vi "test_afis.vi"() -> ()   [LabVIEW 2009]
uses:
  <vilib>/Platform/portaccess.llb/Out Port8.vi
panel:
  out "Numeric":u8
  in  "stop":bool
  # "Numar aleator trimis la portul \n                    8888"
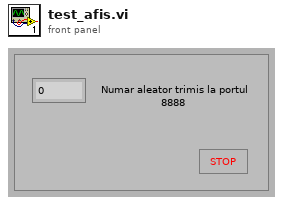
[diagram p1: front panel]
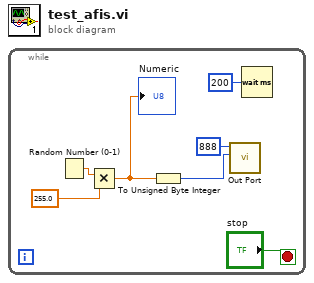
[diagram p0: block diagram]
diagram:
  n1 = while {
    stop <- "stop" stop-if-true
    n2 = Random Number (0-1)() -> (number: 0 to 1=w6:dbl)
    n3 = Multiply(x=w6, y=255.0) -> (x*y=w1:dbl)
    "Numeric" <- w1
    n4 = To Unsigned Byte Integer(number=w1) -> (unsigned 8bit integer=w2:u8)
    n5 = call-poly <vilib>:"Out Port.vi"("write value"=w2, "address"=i16 888) -> ()  [unwired: 7 in, 1 out]
    n6 = Wait (ms)(milliseconds to wait=u32 200) -> ()  [unwired: 1 out]
  }
